vi "GVSView Pic WAIT GRAPH VI.vi"(10 "vi reference":refnum<vi>, 11 "sAction":string) -> (1 "sData_Out":string)   [LabVIEW 2013]
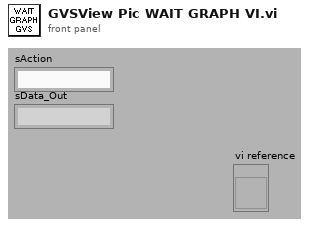
[diagram p1: front panel]
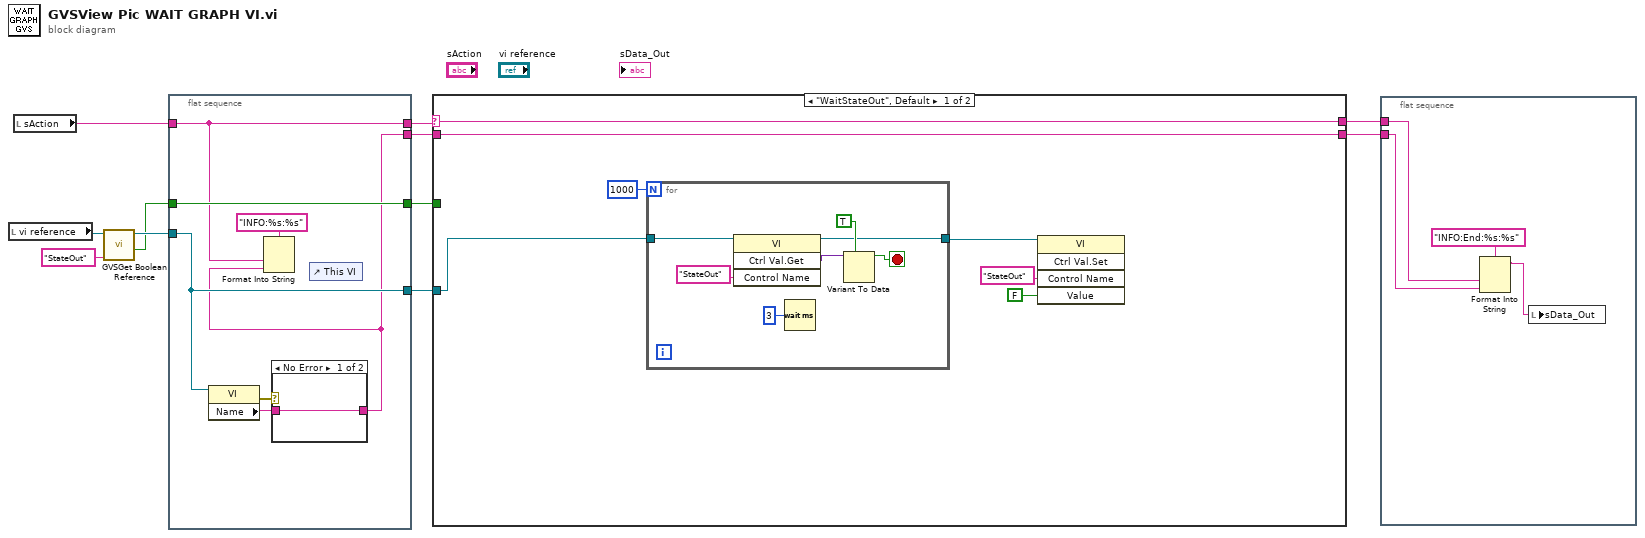
[diagram p0: block diagram]
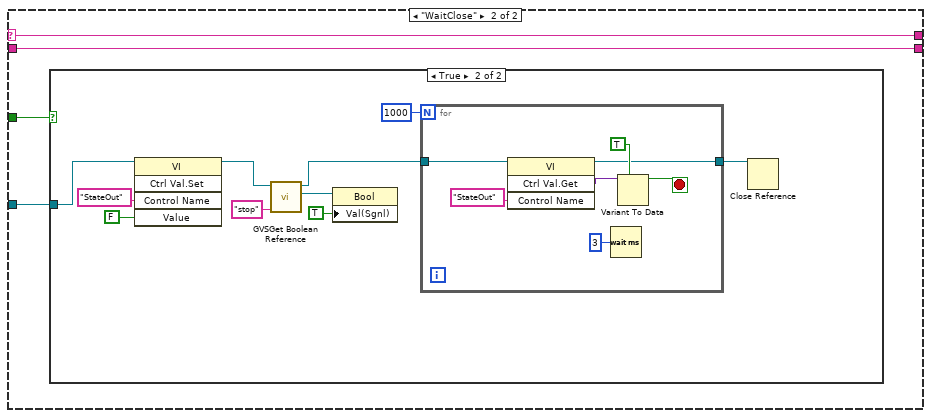
[diagram p2: hidden frame]
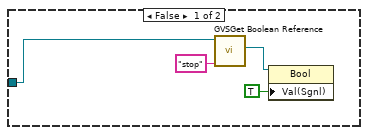
[diagram p3: hidden frame]
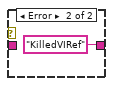
[diagram p4: hidden frame]
diagram:
  n1 = local read "vi reference"() -> (w6:refnum<vi>)
  n2 = local read "sAction"() -> (w5:string)
  n3 = call "GVSGet Boolean Reference.vi"("Label Name"="StateOut", "VI Refnum"=w6) -> ("Boolean"=w9:bool, "VI Refnum Out"=w10:refnum<vi>)  [unwired: 7 in, 1 out]
  n4 = flat-sequence {
    tunnel: [w14] -> w8
    tunnel: w10 -> [w14]
    tunnel: [w18] -> w7
    tunnel: w9 -> [w18]
    tunnel: w5 -> [w13]
    tunnel: [w13] -> w4
    tunnel: [w12] -> w2
    frame #0 {
      n5 = property class="VI"(reference=w14) -> (error out=w16:errorcluster, "Name"=w15:string)  [unwired: 1 in, 1 out]
      n6 = case shown="No Error" w16 {
        tunnel: w15 -> [w19 _]
        tunnel: [w19 "KilledVIRef" ("sAction")] -> w12
        frame No Error {
        }
        frame Error {
        }
      }
      n7 = Format Into String(format string="INFO:%s:%s" ("string"), w13, w12) -> ()  [unwired: 2 in, 2 out]
      n8 = control-ref of="This VI"() -> ()  [unwired: 1 out]
    }
  }
  n9 = case shown="\"WaitStateOut\", Default" w4 {
    selector: w4 -> [w27 w36]
    tunnel: w8 -> [w26 w38]
    tunnel: w7 -> [_ w37]
    tunnel: [w27 w36] -> w3
    tunnel: w2 -> [w25 w35]
    tunnel: [w25 w35] -> w1
    frame "WaitStateOut", Default {
      n10 = for {
        N: 1000 -> [_]
        tunnel: w26 -> [w33]
        tunnel: [w29] -> w22
        stop <- w28 stop-if-true
        n11 = invoke class="VI" method="Ctrl Val.Get"(reference=w33, "Control Name"="StateOut") -> (reference out=w29:refnum<vi>, "Get Control Value Variant"=w32:variant)  [unwired: 2 in, 2 out]
        n12 = Wait (ms)(milliseconds to wait=u32 3) -> ()  [unwired: 1 out]
        n13 = Variant To Data(type=TRUE, Variant=w32) -> (data=w28:bool)  [unwired: 1 in, 1 out]
      }
      n14 = invoke class="VI" method="Ctrl Val.Set"(reference=w22, "Control Name"="StateOut", "Value"=FALSE) -> ()  [unwired: 2 in, 5 out]
    }
    frame "WaitClose" {
      n15 = case shown="True" w37 {
        tunnel: w38 -> [w39 w45]
        frame False {
          n16 = call "GVSGet Boolean Reference.vi"("Label Name"="stop", "VI Refnum"=w39) -> ("Boolean Ref"=w42:refnum<vi>)  [unwired: 7 in, 2 out]
          n17 = property class="Bool"(reference=w42, "Val(Sgnl)"=TRUE) -> ()  [unwired: 1 in, 2 out]
        }
        frame True {
          n18 = invoke class="VI" method="Ctrl Val.Set"(reference=w45, "Control Name"="StateOut", "Value"=FALSE) -> (reference out=w47:refnum<vi>)  [unwired: 2 in, 4 out]
          n19 = call "GVSGet Boolean Reference.vi"("Label Name"="stop", "VI Refnum"=w47) -> ("Boolean Ref"=w50:refnum<vi>, "VI Refnum Out"=w46:refnum<vi>)  [unwired: 7 in, 1 out]
          n20 = property class="Bool"(reference=w50, "Val(Sgnl)"=TRUE) -> ()  [unwired: 1 in, 2 out]
          n21 = for {
            N: 1000 -> [_]
            tunnel: w46 -> [w58]
            tunnel: [w54] -> w44
            stop <- w53 stop-if-true
            n22 = invoke class="VI" method="Ctrl Val.Get"(reference=w58, "Control Name"="StateOut") -> (reference out=w54:refnum<vi>, "Get Control Value Variant"=w57:variant)  [unwired: 2 in, 2 out]
            n23 = Wait (ms)(milliseconds to wait=u32 3) -> ()  [unwired: 1 out]
            n24 = Variant To Data(type=TRUE, Variant=w57) -> (data=w53:bool)  [unwired: 1 in, 1 out]
          }
          n25 = Close Reference(reference=w44) -> ()  [unwired: 1 in, 1 out]
        }
      }
    }
  }
  n26 = flat-sequence {
    tunnel: w3 -> [w62]
    tunnel: w1 -> [w61]
    frame #0 {
      n27 = Format Into String(format string="INFO:End:%s:%s" ("string"), w62, w61) -> (resulting string=w60:string)  [unwired: 2 in, 1 out]
      n28 = local write "sData_Out"(w60) -> ()
    }
  }
